vi "2 PolarPlot.vi"() -> (2 "Velocity":dbl)   [LabVIEW 2011]
panel:
  in  "Boat Angle":dbl
  in  "Wind Vector":cluster{"Wind R":dbl, "Wind Theta":dbl}
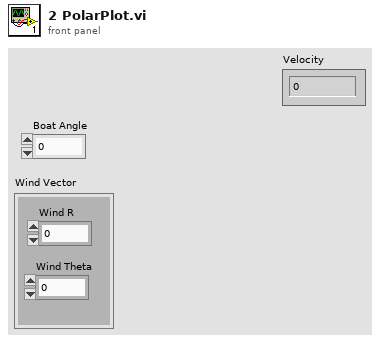
[diagram p1: front panel]
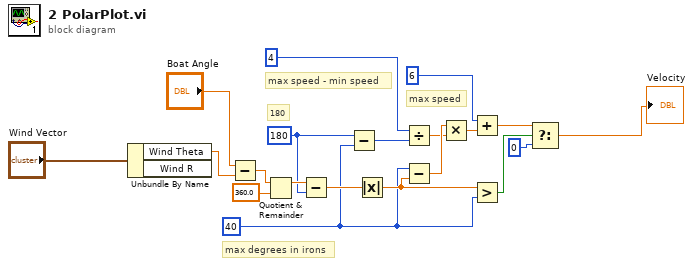
[diagram p0: block diagram]
diagram:
  w7 = 40
  w8 = 180
  # "max speed - min speed"
  # "max speed"
  # "max degrees in irons"
  # "180"
  n1 = Unbundle By Name("Wind Vector") -> ("Wind Theta"=w20:dbl)  [unwired: 1 out]
  n2 = Subtract(x="Boat Angle", y=w20) -> (x-y=w17:dbl)
  n3 = Quotient & Remainder(x=w17, y=360.0) -> (x-y*floor(x/y)=w15:dbl)  [unwired: 1 out]
  n4 = Subtract(x=w15, y=w8) -> (x-y=w14:dbl)
  n5 = Subtract(x=w8, y=w7) -> (x-y=w6:i32)
  n6 = Absolute Value(x=w14) -> (abs(x)=w10:dbl)
  n7 = Divide(x=4, y=w6) -> (x/y=w4:dbl)
  n8 = Subtract(x=w7, y=w10) -> (x-y=w5:dbl)
  n9 = Multiply(x=w5, y=w4) -> (x*y=w3:dbl)
  n10 = Add(x=6, y=w3) -> (x+y=w1:dbl)
  n11 = Greater?(x=w10, y=w7) -> (0:w13:bool)
  n12 = Select(t=w1, s=w13, f=0) -> (s? t:f=→"Velocity":dbl)
